vi "Autonomous Independent.vi"() -> ()   [LabVIEW 2016]
doc: "This VI is called when autonomous begins, and will automatically be terminated when autonomous ends. You can carry out timed or sensor driven robot movement independently without needing to return to the caller."
uses:
  <vilib>/Rock Robotics/WPI/ThirdParty/CanMotor/TalonSRX/WPI_CANTalonSRX_APIFeedbackSelect.ctl
  <vilib>/Rock Robotics/WPI/ThirdParty/CanMotor/TalonSRX/WPI_CANTalonSRX_APIControlMode.ctl
  <vilib>/Rock Robotics/WPI/ThirdParty/CanMotor/TalonSRX/WPI_CANTalonSRX_BrakeOverride.ctl
  <vilib>/Rock Robotics/WPI/Utilities/WPI_GetSetVariantRefNum.vi
  <vilib>/Rock Robotics/Network Tables/NT Read String.vi
  Robot Global Data.vi
  <vilib>/Rock Robotics/Network Tables/NT Write Numeric Array.vi
panel:
  in  "Ramp Rate":dbl format="%#_13g"
  in  "I Zone":dbl format="%#_13g"
  in  "F":dbl=0.005212 format="%#_13g"
  in  "D":dbl format="%#_13g"
  in  "I":dbl format="%#_13g"
  in  "P":dbl=0.5 format="%#_13g"
  in  "Output":dbl
  out "Output":cluster{"Sensor Velocity":dbl, dbl, dbl}(graph)
  # "Be sure to right-click and choose Data Operations>>Make Current Value default if you want to save the array values with the VI"
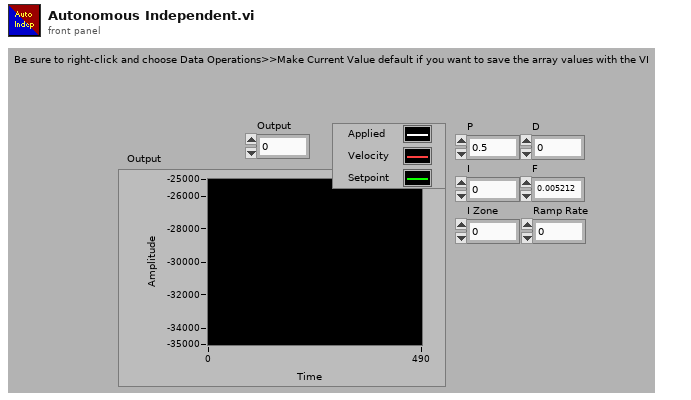
[diagram p1: front panel]
types:
  T1 = typedef "WPI_JoystickDevRef.ctl" = cluster{"Device":T2}
  T2 = typedef "WPI_JoystickDeviceEnum.ctl" = enum16{"USB 0", "USB 1", "USB 2", "USB 3", "USB 4", "USB 5"}
  T3 = typedef "WPI_CANTalonSRX_BrakeOverride.ctl" = enum8{"No Override", "Override to Coast", "Override to Brake"}
  T4 = typedef "WPI_CANTalonSRX_APIControlMode.ctl" = enum8{"Percent VBus", "Speed", "Position", "Slave", "Unchanged / Invalid", "Voltage Compensation", "Current", "Motion Profile", "Motion Magic"}
  T5 = typedef "WPI_CANTalonSRX_APIFeedbackSelect.ctl" = enum16{"Digital Quadrature Encoder", "Analog Potentiometer", "Analog Encoder", "Count on Quad-A (Rising-Edge)", "Count on Quad-A (Falling-Edge)", "CTR Magnetic Enc (Absolute)", "CTR Magnetic Enc (Relative)", "Pulse Width"}
  T6 = typedef "WPI_MotorControlDeviceRef.ctl" = cluster{"DeviceStatus":errorcluster, "Type":T7, "PWM":cluster{"PWM Channel":T8, "DeadBand":T9}, "CAN":cluster{"Device Number":u8, "SetOutput VI Ref":variant, "GetOutput VI Ref":variant, "Enable VI Ref":variant, "Disable VI Ref":variant, "Data":variant}, "Invert":bool}
  T7 = typedef "WPI_MotorControlType.ctl" = enum16{"PWM", "CAN"}
  T8 = typedef "FPGA_DIOPWMChannel.ctl" = enum8{"PWM 0", "PWM 1", "PWM 2", "PWM 3", "PWM 4", "PWM 5", "PWM 6", "PWM 7", "PWM 8", "PWM 9", "PWM MXP 0", "PWM MXP 1", "PWM MXP 2", "PWM MXP 3", "PWM MXP 4", "PWM MXP 5", "PWM MXP 6", "PWM MXP 7", "PWM MXP 8", "PWM MXP 9", "Invalid"}
  T9 = typedef "WPI_PWMDeadband.ctl" = cluster{"Name":string, "maxPositivePwm":i32, "minPositivePwm":i32, "centerPwm":i32, "maxNegativePwm":i32, "minNegativePwm":i32, "angularRange":u16}
  T10 = typedef "WPI_CANTalonSRX_GlobalStatus.ctl" = cluster{"Applied Throttle":dbl, "Module Enabled":bool, "CAN Error":errorcluster, "Closed Loop Error":dbl, "Forward Limit Switch Closed":bool, "Reverse Limit Switch Closed":bool, "Sensor Position":dbl, "Sensor Velocity":dbl, "Current":dbl, "Sticky Fault - Over Temp":bool, "Sticky Fault - Under Voltage":bool, "Sticky Fault - Forward Limit":bool, "Sticky Fault - Reverse Limit":bool, "Sticky Fault - Forward Soft Limit":bool, "Sticky Fault - Reverse Soft Limit":bool, "Brake is Enabled":bool, "Encoder Position":dbl, "Encoder Velocity":dbl, "Encoder Index Count":dbl, "Encoder A Pin State":bool, "Encoder B Pin State":bool, "Encoder Index Pin State":bool, "Analog In":dbl, "Analog In Velocity":dbl, "Temperature (C)":dbl, "Battery Voltage":dbl, "Control 5 Is Supported":bool, "Current Profile Slot Select":dbl, "Pos Div 8":bool, "Vel Div 4":bool, "Pulse Width Position":i32, "Pulse Width Velocity":i32, "Pulse Width Rise To Rise (us)":i32, "Pulse Width Rise To Fall (us)":i32, "Mot Prof Active Is Under Run":bool, "Mot Prof Active Has Under Run":bool, "Mot Prof Active Is Last":bool, "Mot Prof Active Velocity Only":bool, "Mot Prof Active Is Valid":bool, "Mot Prof Buffer Is Full":bool, "Mot Prof Active Profile Slot Select":i32, "Mot Prof NextID":i32, "Mot Prof Count":i32, "Mot Prof Active Velocity":dbl, "Mot Prof Active Position":dbl, "Mot Prof Output Enable":i32}
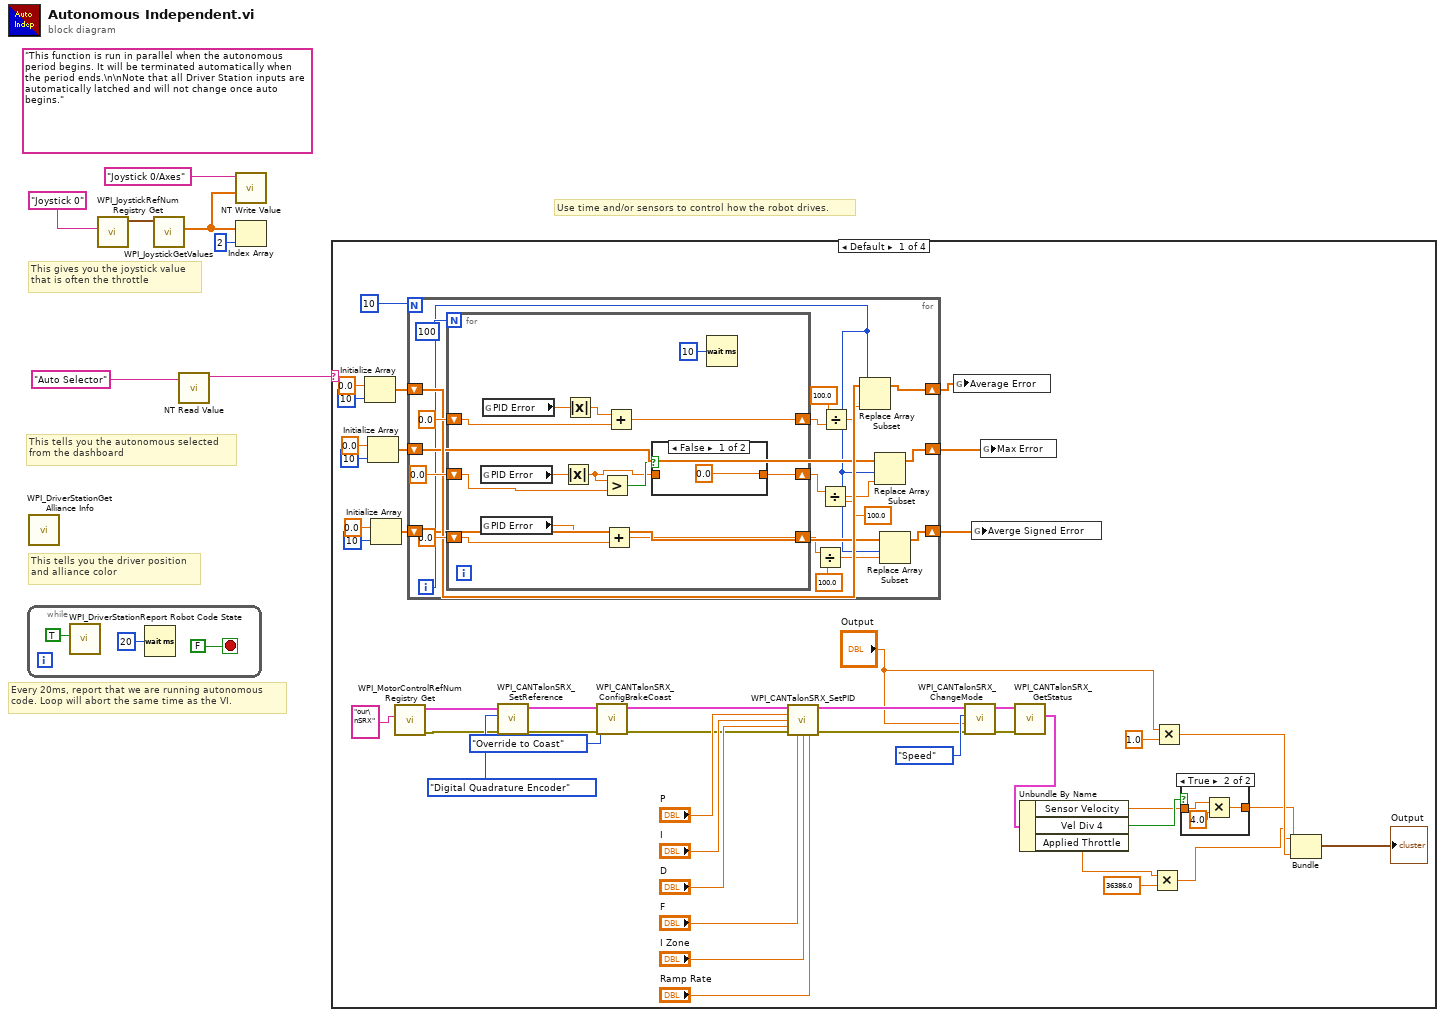
[diagram p0: block diagram]
diagram:
  (unwired) "This function is run in parallel when the autonomous period begins. It will be terminated automatically when the period ends.\n\nNote that all Driver Station inputs are automatically latched and will not change once auto begins."
  # "This tells you the autonomous selected\nfrom the dashboard"
  # "Every 20ms, report that we are running autonomous\ncode. Loop will abort the same time as the VI."
  # "This gives you the joystick value\nthat is often the throttle"
  # "Use time and/or sensors to control how the robot drives."
  # "This tells you the driver position\nand alliance color"
  n1 = while {
    stop <- FALSE stop-if-true
    n2 = call <vilib>:"WPI_DriverStationReport Robot Code State.vi"("Autonomous"=TRUE) -> ()  [unwired: 10 in, 1 out]
    n3 = Wait (ms)(milliseconds to wait=u32 20) -> ()  [unwired: 1 out]
  }
  n4 = call <vilib>:"WPI_DriverStationGet Alliance Info.vi"() -> ()  [unwired: 12 out]
  n5 = call <vilib>:"WPI_JoystickRefNum Registry Get.vi"("refnum name"="Joystick 0") -> ("JoystickDevRef"=w6:T1)  [unwired: 1 in, 9 out]
  n6 = call <vilib>:"WPI_JoystickGetValues.vi"("JoystickDevRef"=w6) -> ("Axes"=w2:dbl[])  [unwired: 6 in, 4 out]
  n7 = call-poly <vilib>:"NT Read Value.vi"("Name"="Auto Selector") -> ("String"=w3:string)  [unwired: 9 in, 1 out]
  n8 = call-poly <vilib>:"NT Write Value.vi"("Numeric Array"=w2, "Name"="Joystick 0/Axes") -> ()  [unwired: 9 in, 1 out]
  n9 = Index Array(array=w2, index=2) -> ()  [unwired: 1 out]
  n10 = case shown="Default" w3 {
    frame Default {
      n11 = Initialize Array(0.0 ("element"), 10 ("dimension size")) -> (w52:dbl[])
      n12 = Initialize Array(0.0 ("element"), 10 ("dimension size")) -> (w46:dbl[])
      n13 = Initialize Array(0.0 ("element"), 10 ("dimension size")) -> (w45:dbl[])
      n14 = call <vilib>:"WPI_MotorControlRefNum Registry Get.vi"("refnum name"="our\nSRX") -> ("error out"=w23:errorcluster, "MotorControlDevRef"=w24:T6)  [unwired: 9 in]
      n15 = for {
        N: 10 -> [_]
        shift-right: [w73] -> w44
        shift-left: w52 -> [w74]
        shift-right: [w72] -> w43
        shift-left: w46 -> [w69]
        shift-right: [w71] -> w42
        shift-left: w45 -> [w70]
        i -> [w68]
        n16 = for {
          N: 100 -> [_]
          shift-right: [w88] -> w67
          shift-left: 0.0 -> [w89]
          shift-right: [w83] -> w64
          shift-left: 0.0 -> [w86]
          shift-right: [w82] -> w61
          shift-left: 0.0 -> [w81]
          n17 = global read "Robot Global Data.vi" "PID Error"() -> (w87:dbl)
          n18 = global read "Robot Global Data.vi" "PID Error"() -> (w80:dbl)
          n19 = global read "Robot Global Data.vi" "PID Error"() -> (w91:dbl)
          n20 = Absolute Value(x=w87) -> (abs(x)=w84:dbl)
          n21 = Absolute Value(x=w91) -> (abs(x)=w90:dbl)
          n22 = Greater?(x=w84, y=w86) -> (0:w85:bool)
          n23 = Add(x=w80, y=w81) -> (x+y=w82:dbl)
          n24 = Add(x=w90, y=w89) -> (x+y=w88:dbl)
          n25 = case shown="False" w85 {
            tunnel: w84 -> [_ w93]
            tunnel: [0.0 w93] -> w83
            frame False {
            }
            frame True {
            }
          }
          n26 = Wait (ms)(milliseconds to wait=u32 10) -> ()  [unwired: 1 out]
        }
        n27 = Divide(x=w61, y=100.0) -> (x/y=w60:dbl)
        n28 = Divide(x=w64, y=100.0) -> (x/y=w62:dbl)
        n29 = Divide(x=100.0, y=w67) -> (x/y=w65:dbl)
        n30 = Replace Array Subset(array=w74, new element=w65, index=w68) -> (w73:dbl[])
        n31 = Replace Array Subset(array=w69, new element=w62, index=w68) -> (w72:dbl[])
        n32 = Replace Array Subset(array=w70, new element=w60, index=w68) -> (w71:dbl[])
      }
      n33 = call <vilib>:"WPI_CANTalonSRX_SetReference.vi"("error in (no error)"=w23, "Feedback Reference"=WPI_CANTalonSRX_APIFeedbackSelect."Digital Quadrature Encoder", "CAN Talon SRX Ref"=w24) -> ("error out"=w30:errorcluster, "CAN Talon SRX Ref"=w31:T6)  [unwired: 7 in]
      n34 = call <vilib>:"WPI_CANTalonSRX_ConfigBrakeCoast.vi"("error in (no error)"=w30, "Brake / Coast Mode"=WPI_CANTalonSRX_BrakeOverride."Override to Coast", "CAN Talon SRX Ref"=w31) -> ("error out"=w28:errorcluster, "CAN Talon SRX Ref"=w29:T6)  [unwired: 7 in]
      n35 = call <vilib>:"WPI_CANTalonSRX_SetPID.vi"("CAN Talon SRX Ref"=w29, "P"="P", "I"="I", "D"="D", "error in (no error)"=w28, "F"="F", "I Zone"="I Zone", "Ramp Rate"="Ramp Rate") -> ("CAN Talon SRX Ref"=w33:T6, "error out"=w32:errorcluster)  [unwired: 6 in]
      n36 = global write "Robot Global Data.vi" "Average Error"(w44) -> ()
      n37 = call <vilib>:"WPI_CANTalonSRX_ChangeMode.vi"("error in (no error)"=w32, "Output"="Output", "Control Mode"=WPI_CANTalonSRX_APIControlMode."Speed", "CAN Talon SRX Ref"=w33) -> ("error out"=w27:errorcluster, "CAN Talon SRX Ref"=w26:T6)  [unwired: 6 in]
      n38 = global write "Robot Global Data.vi" "Averge Signed Error"(w42) -> ()
      n39 = global write "Robot Global Data.vi" "Max Error"(w43) -> ()
      n40 = call <vilib>:"WPI_CANTalonSRX_GetStatus.vi"("error in (no error)"=w27, "CAN Talon SRX Ref"=w26) -> ("Talon SRX Status"=w25:T10)  [unwired: 7 in, 2 out]
      n41 = Unbundle By Name(w25) -> ("Sensor Velocity"=w20:dbl, "Vel Div 4"=w21:bool, "Applied Throttle"=w17:dbl)
      n42 = Multiply(x=w17, y=36386.0) -> (x*y=w13:dbl)
      n43 = Multiply(x="Output", y=1.0) -> (x*y=w14:dbl)
      n44 = case shown="True" w21 {
        tunnel: w20 -> [w55 w57]
        tunnel: [w55 w58] -> w12
        frame False {
        }
        frame True {
          n45 = Multiply(x=w57, y=4.0) -> (x*y=w58:dbl)
        }
      }
      n46 = Bundle(w13, "Sensor Velocity"=w12, w14) -> (→"Output":cluster{dbl, "Sensor Velocity":dbl, dbl})  [unwired: 1 in]
    }
    frame "Alternative 1" {
      # "This sample code describes robot movements in an array. You can extend it to control other motors\non your robot. You can also use file I/O to move the data to a text file."
    }
    frame "Alternative 2" {
    }
    frame "Your Turn" {
    }
  }
